vi "Configure Trigger (Edge).vi"(0 "VISA resource name":refnum<visa-resource-name>, 1 "Trigger Slope (0: Positive)":u16(ring) items=["Positive", "Negative", "Window"], 2 "Trigger Source (1: Channel 1)":u16(ring)=1 items=["Channel 1"=1, "Channel 2"=2, "Channel 3"=3, "Channel 4"=4, "Ext"=5, "Ext5"=6, "AC Line"=7], 5 "Trigger Level (0.0 V)":dbl, 9 "Holdoff Type (0: Time)":u16(ring) items=["TI"], 11 "error in (no error)":errorcluster, 12 "Holdoff Value  (100 ns)":dbl=1e-07) -> (4 "VISA resource name out":refnum<visa-resource-name>, 15 "error out":errorcluster)   [LabVIEW 2021, in "Siglent SDS 1000 2000 Series.lvlib"]
doc: "Configures edge trigger settings. An edge trigger occurs when the trigger signal passes through the voltage threshold that you specify with the Level control and has the slope that you specify with the Slope control."
uses:
  <instrlib>/Siglent SDS 1000 2000 Series/Siglent SDS 1000 2000 Series.lvlib
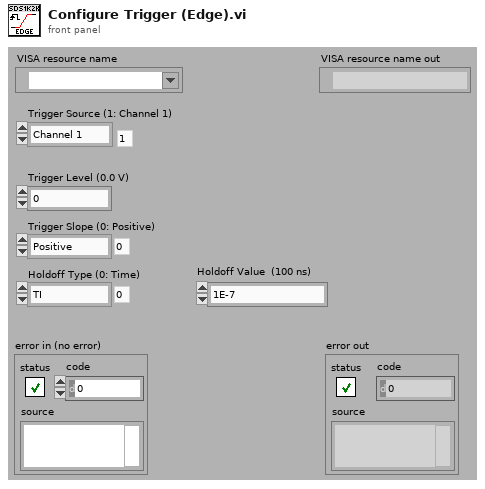
[diagram p1: front panel]
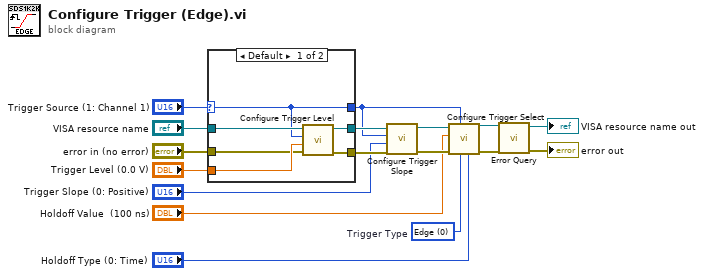
[diagram p0: block diagram]
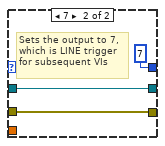
[diagram p2: hidden frame]
diagram:
  w3 = u16 0 items=["Edge", "Dropout", "Glitch", "Interval", "Std", "Sng", "State Qualify", "Edge Qualify"]  # Trigger Type
  n1 = case shown="Default" "Trigger Source (1: Channel 1)" {
    selector: "Trigger Source (1: Channel 1)" -> [w18 _]
    tunnel: "Trigger Level (0.0 V)" -> [w21 _]
    tunnel: [w23 w26] -> w16
    tunnel: [w22 w25] -> w15
    tunnel: "VISA resource name" -> [w20 w26]
    tunnel: "error in (no error)" -> [w19 w25]
    tunnel: [w18 7] -> w4
    frame Default {
      n2 = call <instrlib>:"Configure Trigger Level.vi"("error in (no error)"=w19, "Trigger Level  (0.0 V)"=w21, "Channel (1: Channel 1)"=w18, "VISA resource name"=w20) -> ("error out"=w22:errorcluster, "VISA resource name out"=w23:refnum<visa-resource-name>)  [unwired: 6 in]
    }
    frame 7 {
      # "Sets the output to 7,\nwhich is LINE trigger\nfor subsequent VIs"
    }
  }
  n3 = call <instrlib>:"Configure Trigger Slope.vi"("error in (no error)"=w15, "Trigger Slope (0: Rising)"="Trigger Slope (0: Positive)", "Channel (1: Channel 1)"=w4, "VISA resource name"=w16) -> ("error out"=w12:errorcluster, "VISA resource name out"=w13:refnum<visa-resource-name>)  [unwired: 6 in]
  n4 = call <instrlib>:"Configure Trigger Select.vi"("Hold Type (0: TI)"="Holdoff Type (0: Time)", "Trigger type"=w3, "Trigger Source (1: Channel 1)"=w4, "error in (no error)"=w12, "Hold Value (100 ns)"="Holdoff Value  (100 ns)", "VISA resource name"=w13) -> ("error out"=w6:errorcluster, "VISA resource name out"=w7:refnum<visa-resource-name>)  [unwired: 4 in]
  n5 = call <instrlib>:"Error Query.vi"("error in (no error)"=w6, "VISA resource name"=w7) -> ("error out"=→"error out":errorcluster, "VISA resource name out"=→"VISA resource name out":refnum<visa-resource-name>)  [unwired: 6 in, 2 out]
